vi "Auto_Drive.vi"(8 "Timer?":bool, 9 "Duration":u32=3500, 10 "distance":dbl=88.0 format="%#_13g", 11 "Drive Effort":dbl=1000.0) -> ()   [LabVIEW 2016]
uses:
  <vilib>/Rock Robotics/WPI/SafetyOutput/WPI_SafetyOutputConfigMenu.ctl
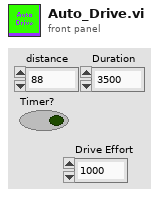
[diagram p1: front panel]
types:
  T1 = typedef "WPI_SafetyOutputConfigMenu.ctl" = enum16{"Enable", "Disable"}
  T2 = typedef "WPI_MotorControlDeviceRef.ctl" = cluster{"DeviceStatus":errorcluster, "Type":T3, "PWM":cluster{"PWM Channel":T4, "DeadBand":T5}, "CAN":cluster{"Device Number":u8, "SetOutput VI Ref":variant, "GetOutput VI Ref":variant, "Enable VI Ref":variant, "Disable VI Ref":variant, "Data":variant}, "Invert":bool}
  T3 = typedef "WPI_MotorControlType.ctl" = enum16{"PWM", "CAN"}
  T4 = typedef "FPGA_DIOPWMChannel.ctl" = enum8{"PWM 0", "PWM 1", "PWM 2", "PWM 3", "PWM 4", "PWM 5", "PWM 6", "PWM 7", "PWM 8", "PWM 9", "PWM MXP 0", "PWM MXP 1", "PWM MXP 2", "PWM MXP 3", "PWM MXP 4", "PWM MXP 5", "PWM MXP 6", "PWM MXP 7", "PWM MXP 8", "PWM MXP 9", "Invalid"}
  T5 = typedef "WPI_PWMDeadband.ctl" = cluster{"Name":string, "maxPositivePwm":i32, "minPositivePwm":i32, "centerPwm":i32, "maxNegativePwm":i32, "minNegativePwm":i32, "angularRange":u16}
  T6 = typedef "WPI_CANTalonSRX_GlobalStatus.ctl" = cluster{"Applied Throttle":dbl, "Module Enabled":bool, "CAN Error":errorcluster, "Closed Loop Error":dbl, "Forward Limit Switch Closed":bool, "Reverse Limit Switch Closed":bool, "Sensor Position":dbl, "Sensor Velocity":dbl, "Current":dbl, "Sticky Fault - Over Temp":bool, "Sticky Fault - Under Voltage":bool, "Sticky Fault - Forward Limit":bool, "Sticky Fault - Reverse Limit":bool, "Sticky Fault - Forward Soft Limit":bool, "Sticky Fault - Reverse Soft Limit":bool, "Brake is Enabled":bool, "Encoder Position":dbl, "Encoder Velocity":dbl, "Encoder Index Count":dbl, "Encoder A Pin State":bool, "Encoder B Pin State":bool, "Encoder Index Pin State":bool, "Analog In":dbl, "Analog In Velocity":dbl, "Temperature (C)":dbl, "Battery Voltage":dbl, "Control 5 Is Supported":bool, "Current Profile Slot Select":dbl, "Pos Div 8":bool, "Vel Div 4":bool, "Pulse Width Position":i32, "Pulse Width Velocity":i32, "Pulse Width Rise To Rise (us)":i32, "Pulse Width Rise To Fall (us)":i32, "Mot Prof Active Is Under Run":bool, "Mot Prof Active Has Under Run":bool, "Mot Prof Active Is Last":bool, "Mot Prof Active Velocity Only":bool, "Mot Prof Active Is Valid":bool, "Mot Prof Buffer Is Full":bool, "Mot Prof Active Profile Slot Select":i32, "Mot Prof NextID":i32, "Mot Prof Count":i32, "Mot Prof Active Velocity":dbl, "Mot Prof Active Position":dbl, "Mot Prof Output Enable":i32}
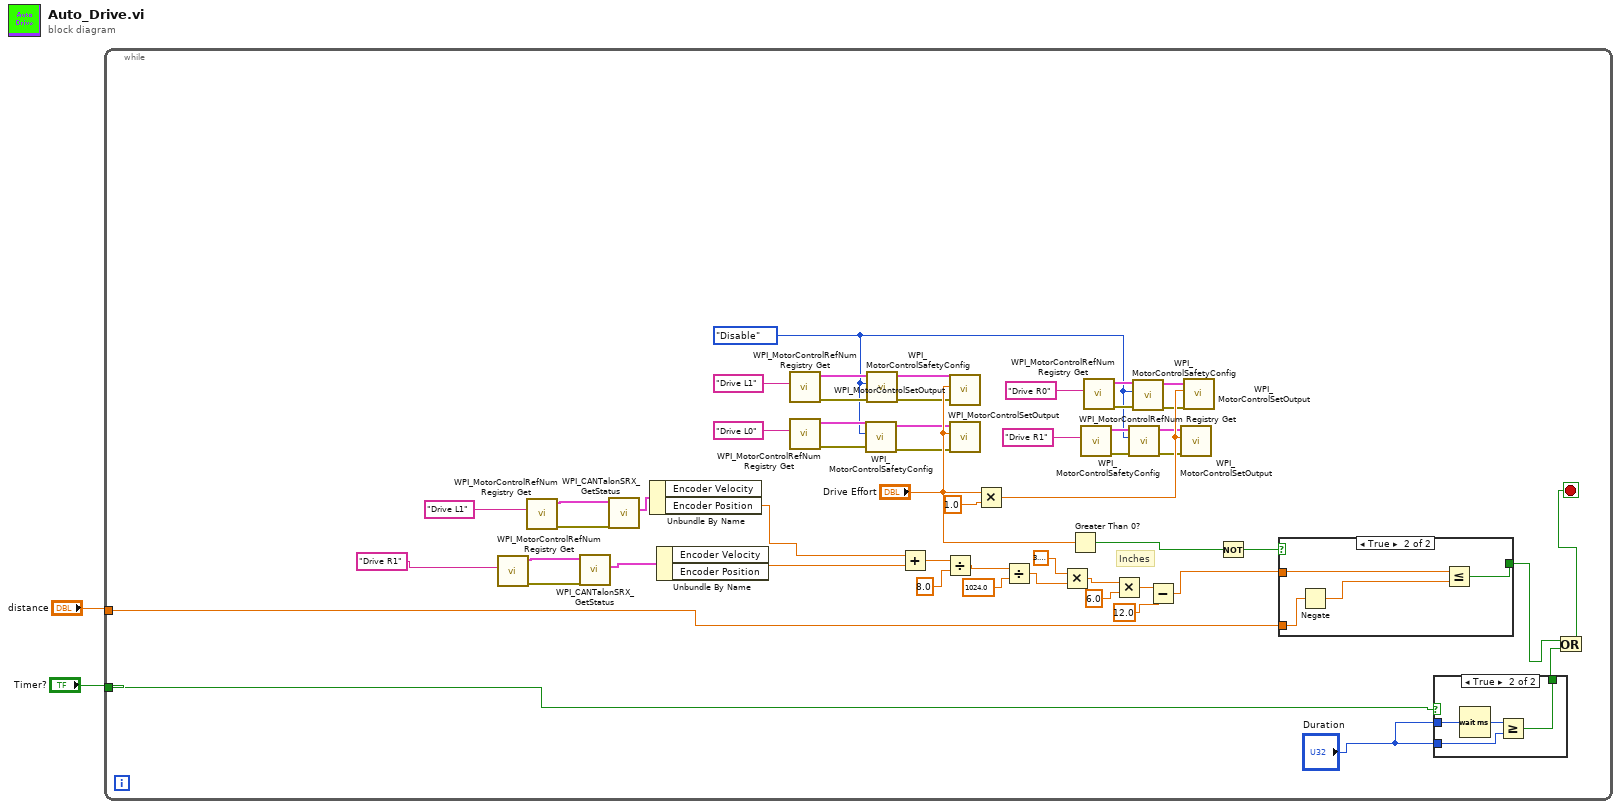
[diagram p0: block diagram]
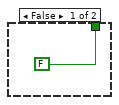
[diagram p2: hidden frame]
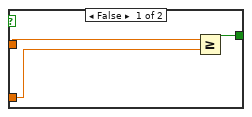
[diagram p3: hidden frame]
diagram:
  n1 = while {
    tunnel: "distance" -> [w36]
    tunnel: "Timer?" -> [w31]
    stop <- w25 stop-if-true
    w4 = WPI_SafetyOutputConfigMenu."Disable" ("mode")
    # "Inches"
    n2 = call <vilib>:"WPI_MotorControlRefNum Registry Get.vi"("refnum name"="Drive R1") -> ("error out"=w51:errorcluster, "MotorControlDevRef"=w52:T2)  [unwired: 9 in]
    n3 = call <vilib>:"WPI_MotorControlRefNum Registry Get.vi"("refnum name"="Drive L1") -> ("error out"=w48:errorcluster, "MotorControlDevRef"=w53:T2)  [unwired: 9 in]
    n4 = call <vilib>:"WPI_CANTalonSRX_GetStatus.vi"("error in (no error)"=w51, "CAN Talon SRX Ref"=w52) -> ("Talon SRX Status"=w49:T6)  [unwired: 7 in, 2 out]
    n5 = call <vilib>:"WPI_CANTalonSRX_GetStatus.vi"("error in (no error)"=w48, "CAN Talon SRX Ref"=w53) -> ("Talon SRX Status"=w50:T6)  [unwired: 7 in, 2 out]
    n6 = Unbundle By Name(w50) -> ("Encoder Position"=w3:dbl)  [unwired: 1 out]
    n7 = Unbundle By Name(w49) -> ("Encoder Position"=w39:dbl)  [unwired: 1 out]
    n8 = call <vilib>:"WPI_MotorControlRefNum Registry Get.vi"("refnum name"="Drive L1") -> ("error out"=w19:errorcluster, "MotorControlDevRef"=w20:T2)  [unwired: 9 in]
    n9 = call <vilib>:"WPI_MotorControlRefNum Registry Get.vi"("refnum name"="Drive L0") -> ("error out"=w15:errorcluster, "MotorControlDevRef"=w16:T2)  [unwired: 9 in]
    n10 = call <vilib>:"WPI_MotorControlSafetyConfig.vi"("error in (no error)"=w15, "mode"=w4, "MotorControlDevRef"=w16) -> ("error out"=w13:errorcluster, "MotorControlDevRef"=w14:T2)  [unwired: 7 in]
    n11 = call <vilib>:"WPI_MotorControlSafetyConfig.vi"("error in (no error)"=w19, "mode"=w4, "MotorControlDevRef"=w20) -> ("error out"=w17:errorcluster, "MotorControlDevRef"=w18:T2)  [unwired: 7 in]
    n12 = Add(x=w3, y=w39) -> (x+y=w47:dbl)
    n13 = Divide(x=w47, y=8.0) -> (x/y=w45:dbl)
    n14 = call <vilib>:"WPI_MotorControlSetOutput.vi"("error in (no error)"=w17, "Output"="Drive Effort", "MotorControlDevRef"=w18) -> ()  [unwired: 6 in, 3 out]
    n15 = call <vilib>:"WPI_MotorControlSetOutput.vi"("error in (no error)"=w13, "Output"="Drive Effort", "MotorControlDevRef"=w14) -> ()  [unwired: 6 in, 3 out]
    n16 = Multiply(x="Drive Effort", y=1.0) -> (x*y=w22:dbl)
    n17 = Divide(x=w45, y=1024.0) -> (x/y=w43:dbl)
    n18 = Multiply(x=3.141592653589793, y=w43) -> (x*y=w41:dbl)
    n19 = Greater Than 0?(x="Drive Effort") -> (x > 0?=w32:bool)
    n20 = call <vilib>:"WPI_MotorControlRefNum Registry Get.vi"("refnum name"="Drive R1") -> ("error out"=w7:errorcluster, "MotorControlDevRef"=w8:T2)  [unwired: 9 in]
    n21 = call <vilib>:"WPI_MotorControlRefNum Registry Get.vi"("refnum name"="Drive R0") -> ("error out"=w11:errorcluster, "MotorControlDevRef"=w12:T2)  [unwired: 9 in]
    n22 = Multiply(x=w41, y=6.0) -> (x*y=w35:dbl)
    n23 = call <vilib>:"WPI_MotorControlSafetyConfig.vi"("error in (no error)"=w7, "mode"=w4, "MotorControlDevRef"=w8) -> ("error out"=w6:errorcluster, "MotorControlDevRef"=w5:T2)  [unwired: 7 in]
    n24 = call <vilib>:"WPI_MotorControlSafetyConfig.vi"("error in (no error)"=w11, "mode"=w4, "MotorControlDevRef"=w12) -> ("error out"=w10:errorcluster, "MotorControlDevRef"=w9:T2)  [unwired: 7 in]
    n25 = Subtract(x=w35, y=12.0) -> (x-y=w33:dbl)
    n26 = call <vilib>:"WPI_MotorControlSetOutput.vi"("error in (no error)"=w6, "Output"=w22, "MotorControlDevRef"=w5) -> ()  [unwired: 6 in, 3 out]
    n27 = call <vilib>:"WPI_MotorControlSetOutput.vi"("error in (no error)"=w10, "Output"=w22, "MotorControlDevRef"=w9) -> ()  [unwired: 6 in, 3 out]
    n28 = Not(x=w32) -> (.not. x?=w23:bool)
    n29 = case shown="True" w23 {
      tunnel: [w61 w67] -> w27
      tunnel: w36 -> [w62 w65]
      tunnel: w33 -> [w63 w64]
      frame False {
        n30 = Greater Or Equal?(x=w63, y=w62) -> (x >= y?=w61:bool)
      }
      frame True {
        n31 = Negate(x=w65) -> (-x=w66:dbl)
        n32 = Less Or Equal?(x=w64, y=w66) -> (x <= y?=w67:bool)
      }
    }
    n33 = case shown="True" w31 {
      tunnel: "Duration" -> [_ w59]
      tunnel: [FALSE w58] -> w26
      tunnel: "Duration" -> [_ w57]
      frame False {
      }
      frame True {
        n34 = Wait (ms)(milliseconds to wait=w57) -> (millisecond timer value=w60:u32)
        n35 = Greater Or Equal?(x=w60, y=w59) -> (x >= y?=w58:bool)
      }
    }
    n36 = Or(x=w27, y=w26) -> (x .or. y?=w25:bool)
  }
